vi "Read States.vi"(8 "error in (no error)":errorcluster, 11 "DefaultPsTactic in":refnum<class "DefaultPsTactic.lvclass">) -> (0 "error out":errorcluster, 2 "States":enum16{"Exit", "AttackPs", "DefensePs"}(ring), 3 "DefaultPsTactic out":refnum<class "DefaultPsTactic.lvclass">)   [LabVIEW 2020, in "DefaultPsTactic.lvclass"]
uses:
  DefaultPsTactic.lvclass
  DefaultPsTactic.lvclass/DefaultPsTactic.ctl
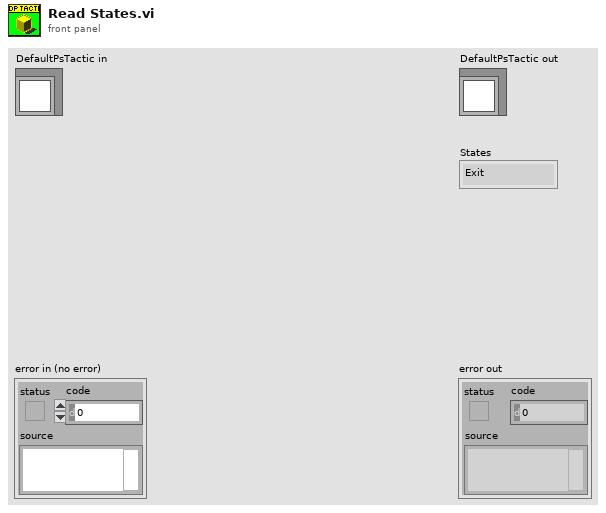
[diagram p1: front panel]
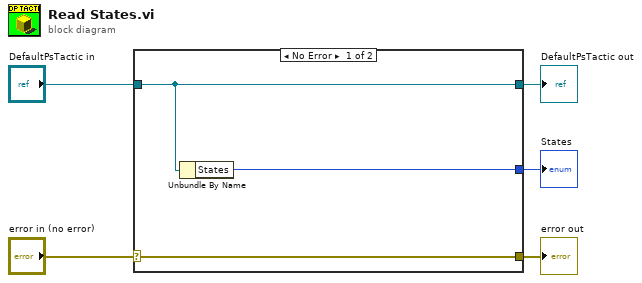
[diagram p0: block diagram]
diagram:
  n1 = case shown="No Error" "error in (no error)" {
    selector: "error in (no error)" -> [w8 w9]
    tunnel: [w8 w9] -> w4
    tunnel: [w7 w10] -> w2
    tunnel: "DefaultPsTactic in" -> [w7 w10]
    tunnel: [w6 _] -> w1
    frame No Error {
      n2 = Unbundle By Name(w7) -> ("States"=w6:enum16{"Exit", "AttackPs", "DefensePs"})
    }
    frame Error {
    }
  }
  "error out" <- w4
  "DefaultPsTactic out" <- w2
  "States" <- w1
